vi "TypeMap FGV.vi"(8 "error in (no error)":errorcluster, 9 "Action":enum16{"Get", "Set"}(ring), 10 "object":refnum<class>, 11 "TypeMap in":refnum<class "TypeMap.lvclass">) -> (0 "error out":errorcluster, 2 "found/replaced?":bool, 3 "TypeMap out":refnum<class "TypeMap.lvclass">)   [LabVIEW 2020, in "ORM.lvlib" / "TypeMap.lvclass"]
uses:
  TypeMap.lvclass
  <userlib>/_OpenG.lib/lvdata/lvdata.llb/openg_variant.lvlib
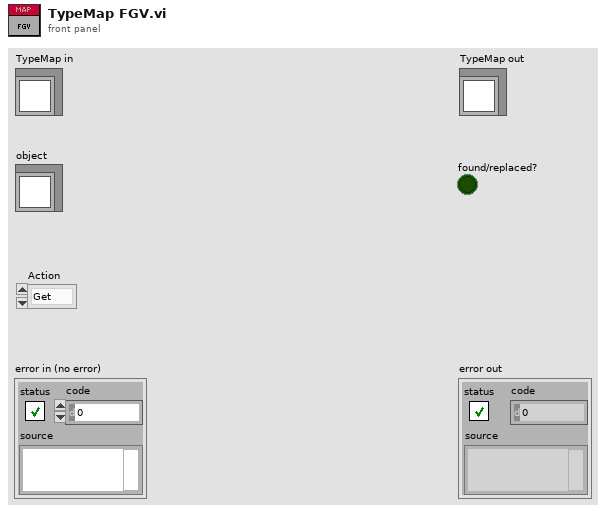
[diagram p1: front panel]
types:
  T1 = map{refnum<class>, refnum<class "TypeMap.lvclass">}
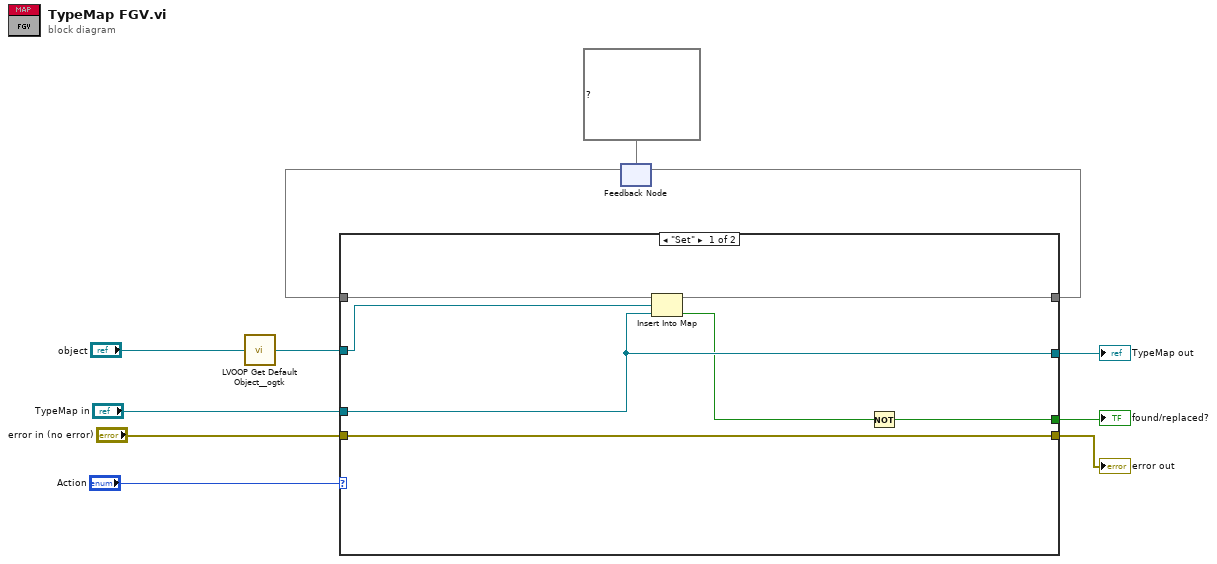
[diagram p0: block diagram]
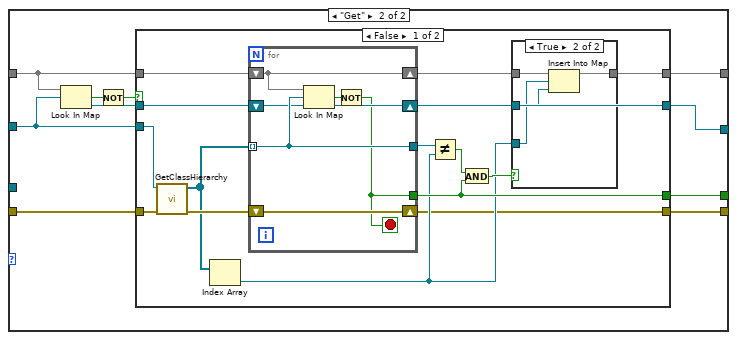
[diagram p2: hidden frame]
diagram:
  n1 = call <userlib>:"LVOOP Get Default Object__ogtk.vi"("Object"="object") -> ("Object Default Instance"=w2:refnum<class>)
  n2 = feedback #1(T1 {} ("map")) -> (w10:T1)
  n3 = case shown="\"Set\"" "Action" {
    tunnel: w10 -> [w17 w19]
    tunnel: [w18 w26] -> w11
    tunnel: w2 -> [w13 w24]
    tunnel: [w14 w28] -> w6
    tunnel: "error in (no error)" -> [w12 w20]
    tunnel: [w16 w27] -> w5
    tunnel: [w12 w25] -> w7
    tunnel: "TypeMap in" -> [w16 _]
    frame "Set" {
      n4 = Insert Into Map(map in=w17, key=w13, value=w16) -> (map out=w18:T1, value unchanged?=w15:bool)  [unwired: 1 out]
      n5 = Not(x=w15) -> (.not. x?=w14:bool)
    }
    frame "Get" {
      n6 = Look In Map(map=w19, key=w24) -> (key not found?=w23:bool, value=w21:refnum<class "TypeMap.lvclass">)  [unwired: 1 in]
      n7 = Not(x=w23) -> (.not. x?=w22:bool)
      n8 = case shown="False" w22 {
        selector: w22 -> [_ w58]
        tunnel: [w41 w58] -> w28
        tunnel: [w39 w59] -> w27
        tunnel: [w38 w56] -> w26
        tunnel: [w29 w57] -> w25
        tunnel: w24 -> [w35 _]
        tunnel: w21 -> [w37 w59]
        tunnel: w20 -> [w34 w57]
        tunnel: w19 -> [w33 w56]
        frame False {
          n9 = call "GetClassHierarchy.vi"("error in (no error)"=w34, "object"=w35) -> ("error out"=w36:errorcluster, "ClassHierarchy"=w32:refnum<class>[])  [unwired: 8 in]
          n10 = Index Array(array=w32) -> (element=w31:refnum<class>)  [unwired: 1 in]
          n11 = for {
            tunnel: [w50] -> w41
            shift-right: [w52] -> w29
            shift-left: w36 -> [w52]
            shift-right: [w53] -> w39
            shift-left: w37 -> [w54]
            tunnel: w32 -> [w55] mode=indexing
            tunnel: [w55] -> w43
            shift-right: [w49] -> w30
            shift-left: w33 -> [w49]
            stop <- w50 stop-if-true
            n12 = Look In Map(map=w49, key=w55, default value=w54) -> (key not found?=w51:bool, value=w53:refnum<class "TypeMap.lvclass">)
            n13 = Not(x=w51) -> (.not. x?=w50:bool)
          }
          n14 = Not Equal?(x=w43, y=w31) -> (x != y?=w42:bool)
          n15 = And(x=w42, y=w41) -> (x .and. y?=w40:bool)
          n16 = case shown="True" w40 {
            tunnel: w31 -> [_ w47]
            tunnel: [w44 w45] -> w38
            tunnel: w39 -> [_ w46]
            tunnel: w30 -> [w44 w48]
            frame False {
            }
            frame True {
              n17 = Insert Into Map(map in=w48, key=w47, value=w46) -> (map out=w45:T1)  [unwired: 2 out]
            }
          }
        }
        frame True {
        }
      }
    }
  }
  "error out" <- w7
  "TypeMap out" <- w5
  "found/replaced?" <- w6
  n18 = feedback-in #1(w11) -> ()
